vi "init.vi"(0 "+3.3VDSupplyTest in":refnum<class "+3.3VDSupplyTest.lvclass">, 1 "Log":refnum<class "ITestLog.lvclass">, 5 "DAQ Channel To Read":refnum<k21>, 7 "Expected Value":dbl[unit], 9 "Tolerance":dbl[unit], 11 "error in (no error)":errorcluster, 12 "Samples To Read":dbl) -> (4 "+3.3VDSupplyTest out":refnum<class "+3.3VDSupplyTest.lvclass">, 15 "error out":errorcluster)   [LabVIEW 2015, in "+3.3VDSupplyTest.lvclass"]
uses:
  +3.3VDSupplyTest.lvclass
  Model/TestLog/ITestLog/ITestLog.lvclass
  +3.3VDSupplyTest.lvclass/+3.3VDSupplyTest.ctl
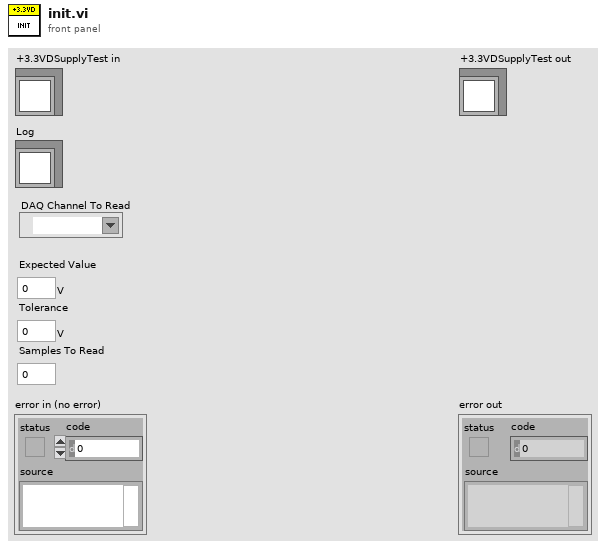
[diagram p1: front panel]
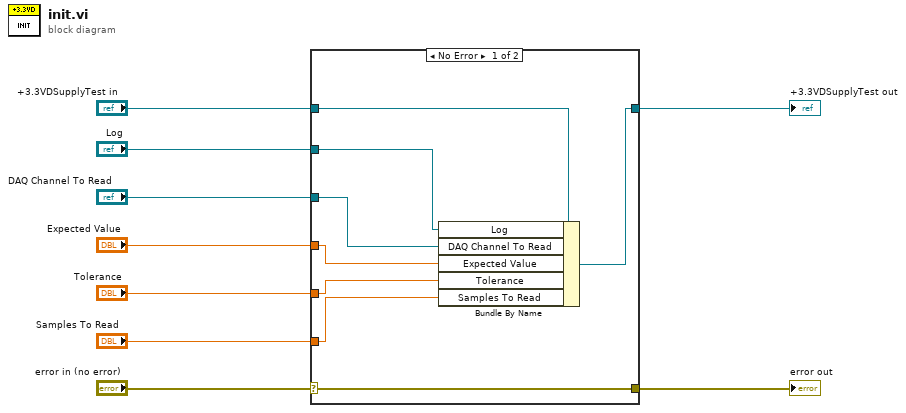
[diagram p0: block diagram]
diagram:
  n1 = case shown="No Error" "error in (no error)" {
    selector: "error in (no error)" -> [w17 w19]
    tunnel: [w17 w19] -> w6
    tunnel: [w15 w18] -> w7
    tunnel: "+3.3VDSupplyTest in" -> [w16 w18]
    tunnel: "Log" -> [w10 _]
    tunnel: "DAQ Channel To Read" -> [w11 _]
    tunnel: "Expected Value" -> [w12 _]
    tunnel: "Tolerance" -> [w13 _]
    tunnel: "Samples To Read" -> [w14 _]
    frame No Error {
      n2 = Bundle By Name(cluster=w16, "Log"=w10, "DAQ Channel To Read"=w11, "Expected Value"=w12, "Tolerance"=w13, "Samples To Read"=w14) -> (w15:refnum<class "+3.3VDSupplyTest.lvclass">)
    }
    frame Error {
    }
  }
  "error out" <- w6
  "+3.3VDSupplyTest out" <- w7
